vi "HFRR ADV v03 new software.vi"() -> ()   [LabVIEW 2025] (continued)
                      n2721 = Fract/Exp String To Number(string=w3763) -> (number=→"AVP 2":dbl)  [unwired: 3 in, 1 out]
                    }
                    frame 12 {
                      n2722 = Fract/Exp String To Number(string=w3765) -> (number=→"HCF 2":dbl)  [unwired: 3 in, 1 out]
                    }
                    frame 13 {
                      n2723 = Fract/Exp String To Number(string=w3767) -> (number=→"WS1.4 2":dbl)  [unwired: 3 in, 1 out]
                    }
                    frame 14, Default {
                    }
                  }
                }
              }
              frame #2 {
              }
            }
            n2724 = local write "OK Button 16"(FALSE ("OK Button 13")) -> ()
          }
        }
        n2725 = Index Array(array=w3411, index="Select Printer 3") -> (element=w3413:string)
        "Selected Printer" <- w3413
        n2726 = case shown="True" w3408 {
          frame False {
          }
          frame True {
            n2727 = flat-sequence {
              frame #0 {
              }
              frame #1 {
                n2728 = Wait (ms)(milliseconds to wait=u32 100) -> ()  [unwired: 1 out]
              }
              frame #2 {
                n2729 = local write "OK Button 16"(FALSE ("Print 3")) -> ()
              }
            }
          }
        }
        n2730 = case shown="True" "Print" {
          tunnel: w3413 -> [_ w3705]
          frame False {
          }
          frame True {
            (unwired) i16 6 ("width (-)")
            (unwired) "TESTED BY : "
            (unwired) "TESTED DATE :"
            (unwired) "SAMPLE ID : "
            (unwired) "SAMPLE DESIGN : "
            w3663 = "\r"
            w3680 = "\r"
            # "add image"
            n2731 = local read "Sample ID"() -> (w3653:string)
            n2732 = local read "Tested by"() -> (w3656:string)
            n2733 = local read "String 34"() -> (w3643:string)
            n2734 = local read "String 45"() -> (w3623:string)
            n2735 = local read "String 35"() -> (w3638:string)
            n2736 = local read "String 37"() -> (w3636:string)
            n2737 = local read "String 32"() -> (w3658:string)
            n2738 = local read "String 36"() -> (w3633:string)
            n2739 = local read "String 31"() -> (w3657:string)
            n2740 = local read "Test Date"() -> (w3654:string)
            n2741 = local read "String 33"() -> (w3659:string)
            n2742 = local read "String 38"() -> (w3629:string)
            n2743 = local read "String 39"() -> (w3626:string)
            n2744 = local write "Print"(FALSE ("Print FF")) -> ()
            n2745 = local read "S 39"() -> (w3641:string)
            n2746 = local read "S 38"() -> (w3648:string)
            n2747 = local read "Temperature before test 2"() -> (w3679:dbl)
            n2748 = local read "Temperature after test 2"() -> (w3669:dbl)
            n2749 = local read "Humidity before test 2"() -> (w3694:dbl)
            n2750 = local read "Humidity after test 2"() -> (w3678:dbl)
            n2751 = local read "MWSD 2"() -> (w3683:dbl)
            n2752 = local read "WS1.4 2"() -> (w3661:dbl)
            n2753 = Concatenate Strings("2)" ("string"), w3643) -> (w3644:string)
            n2754 = Concatenate Strings("3)" ("string"), w3641) -> (w3642:string)
            n2755 = Concatenate Strings("1)" ("string"), w3648) -> (w3647:string)
            n2756 = Concatenate Strings("4)" ("string"), w3638) -> (w3639:string)
            n2757 = Concatenate Strings("5)" ("string"), w3636) -> (w3635:string)
            n2758 = Concatenate Strings("6)" ("string"), w3633) -> (w3632:string)
            n2759 = Concatenate Strings("7)" ("string"), w3629) -> (w3630:string)
            n2760 = Concatenate Strings("8)" ("string"), w3626) -> (w3627:string)
            n2761 = local read "HCF 2"() -> (w3665:dbl)
            n2762 = local read "AVP 2"() -> (w3682:dbl)
            n2763 = local read "s.NO"() -> (w3624:string)
            n2764 = call <vilib>:"New Report.vi"("report type"=enum16{"Standard Report", "HTML"}."Standard Report") -> ("report out"=w3703:refnum<class "NI_report.lvclass">, "error out"=w3702:errorcluster)  [unwired: 13 in]
            n2765 = local read "TITTLE"() -> (w3655:string)
            n2766 = Concatenate Strings(w3680, w3623, w3624, w3680, w3658, w3653, w3680, w3657, w3654, w3680, w3659, w3656, w3680) -> (w3673:string)
            "test by" <- w3673
            n2767 = Number To Fractional String(number=w3679, width (-)=i16 6, precision (6)=i16 2) -> (F-format string=w3668:string)  [unwired: 1 in]
            n2768 = Number To Fractional String(number=w3678, width (-)=i16 6, precision (6)=i16 2) -> (F-format string=w3681:string)  [unwired: 1 in]
            n2769 = Number To Fractional String(number=w3694, width (-)=i16 6, precision (6)=i16 2) -> (F-format string=w3699:string)  [unwired: 1 in]
            n2770 = Number To Fractional String(number=w3683, width (-)=i16 6, precision (6)=i16 2) -> (F-format string=w3685:string)  [unwired: 1 in]
            n2771 = Number To Fractional String(number=w3669, width (-)=i16 6, precision (6)=i16 2) -> (F-format string=w3670:string)  [unwired: 1 in]
            n2772 = Number To Fractional String(number=w3682, width (-)=i16 6, precision (6)=i16 2) -> (F-format string=w3684:string)  [unwired: 1 in]
            n2773 = Number To Fractional String(number=w3665, width (-)=i16 6, precision (6)=i16 2) -> (F-format string=w3664:string)  [unwired: 1 in]
            n2774 = Number To Fractional String(number=w3661, precision (6)=i16 2) -> (F-format string=w3660:string)  [unwired: 2 in]
            n2775 = call-dynamic "Set Report Header Text.vi"("report in"=w3703, "center header text"=w3655, "error in (no error)"=w3702) -> ("report out"=w3674:refnum<class "NI_report.lvclass">, "error out"=w3675:errorcluster)  [unwired: 11 in]
            n2776 = Concatenate Strings(w3663, w3647, w3699, w3663, w3644, w3668, w3663, w3642, w3681, w3663, w3639, w3670, w3663, w3635, w3685, w3663, w3632, w3684, w3663, w3630, w3664, w3663, w3627, w3660) -> (w3651:string)
            "export 2" <- w3651
            n2777 = call-poly <vilib>:"Append Report Text.vi"("report in"=w3674, "text"=w3673, "error in (no error)"=w3675) -> ("report out"=w3677:refnum<class "NI_report.lvclass">, "error out"=w3676:errorcluster)  [unwired: 9 in, 2 out]
            n2778 = local read "test by"() -> (w3650:string)
            n2779 = local read "TITTLE"() -> (w3652:string)
            n2780 = call-poly <vilib>:"Append Report Text.vi"("report in"=w3677, "error in (no error)"=w3676) -> ("report out"=w3698:refnum<class "NI_report.lvclass">, "error out"=w3696:errorcluster)  [unwired: 10 in, 2 out]
            n2781 = Concatenate Strings(w3652, w3651, w3650) -> (→"output":string)
            n2782 = call-poly <vilib>:"Append Report Text.vi"("report in"=w3698, "text"=w3651, "error in (no error)"=w3696) -> ("report out"=w3697:refnum<class "NI_report.lvclass">, "error out"=w3695:errorcluster)  [unwired: 9 in, 2 out]
            n2783 = call-dynamic "Print Report.vi"("report in"=w3697, "printer name (default)"=w3705, "error in (no error)"=w3695) -> ("report out"=w3707:refnum<class "NI_report.lvclass">, "error out"=w3708:errorcluster)  [unwired: 11 in]
            n2784 = call-dynamic "Dispose Report.vi"("report in"=w3707, "error in (no error)"=w3708) -> ()  [unwired: 13 in, 1 out]
          }
        }
        n2785 = case shown="True" "Print 2" {
          frame False {
          }
          frame True {
            n2786 = flat-sequence {
              frame #0 {
                n2787 = local read "s.NO"() -> (→"s.NO 2":string)
                n2788 = Wait (ms)(milliseconds to wait=u32 20) -> ()  [unwired: 1 out]
                n2789 = local read "Sample ID  3"() -> (→"Sample ID  6":string)
                n2790 = local read "Sample ID  4"() -> (→"Sample ID  7":string)
                n2791 = local read "Sample ID"() -> (→"Sample ID  2":string)
                n2792 = local read "Tested by"() -> (→"Tested by 2":string)
                n2793 = local read "Test Date"() -> (→"Test Date 2":string)
                n2794 = local read "Humidity after test 3"() -> (→"Humidity after test 4":dbl)
                n2795 = local read "Ref A Test Date :"() -> (→"TITTLE 4":string)
                n2796 = local read "Temperature before test 3"() -> (w3530:dbl)
                n2797 = local read "Temperature before test 3"() -> (→"Temperature after test 5":dbl)
                n2798 = local read "Temperature after test 3"() -> (→"Temperature after test 4":dbl)
                n2799 = local read "Humidity before test 3"() -> (→"Humidity before test 4":dbl)
                n2800 = local write "Temperature before test 3"(w3530) -> ()
                n2801 = local read "image data"() -> (w3521:T11)
                n2802 = String To Path(string="C:\\LAB-IQ\\im\\Temp_resized.jpg") -> (path=w3522:path)
                "path 2" <- w3522
                n2803 = call <vilib>:"Write JPEG File.vi"("image data"=w3521, "path to JPEG file"=w3522) -> ()  [unwired: 8 in, 2 out]
                "Ref A Test Date :" <- "Ref A Test Date :"
                "Ref B Test Date :" <- "Ref B Test Date :"
                "Ref B Scar Value :" <- "Ref B Scar Value :"
                "Ref A Scar Value :" <- "Ref A Scar Value :"
              }
              frame #1 {
                (unwired) HTML_Report_Image_Alignment."MIDDLE" ("alignment (default)")
                w3558 = u16 0 items=["portrait", "landscape"] ("orientation (portrait)")
                (unwired) HTML_Report_Image_Alignment."ABSMIDDLE" ("alignment (default)")
                (unwired) "TESTED BY : "
                (unwired) "TESTED DATE :"
                (unwired) "SAMPLE ID : "
                (unwired) "SAMPLE DESIGN : "
                w3591 = "\r"
                # "add image"
                n2804 = Wait (ms)(milliseconds to wait=u32 20) -> ()  [unwired: 1 out]
                n2805 = local read "Sample ID  2"() -> (w3584:string)
                n2806 = local read "Wear Scar X"() -> (w3556:dbl)
                "Length ( microns ) 2" <- w3556
                n2807 = local read "Wear Scar Y"() -> (w3555:dbl)
                "Wear Scar Y ( microns ) :" <- w3555
                n2808 = local read "Test Date 2"() -> (w3585:string)
                n2809 = local read "Tested by 2"() -> (w3586:string)
                n2810 = local read "String 46"() -> (w3582:string)
                n2811 = local read "String 48"() -> (w3588:string)
                n2812 = local read "String 47"() -> (w3587:string)
                n2813 = local read "String 49"() -> (w3589:string)
                n2814 = local read "String 10"() -> (w3542:string)
                n2815 = local read "s.NO 2"() -> (w3583:string)
                n2816 = Add(x=w3556, y=w3555) -> (x+y=w3554:dbl)
                n2817 = call <vilib>:"New Report.vi"("report type"=enum16{"Standard Report", "HTML"}."HTML") -> ("report out"=w3562:refnum<class "NI_report.lvclass">, "error out"=w3560:errorcluster)  [unwired: 13 in]
                n2818 = Concatenate Strings(w3591, w3582, w3583, w3591, w3588, w3584, w3591, w3587, w3585, w3591, w3589, w3586, w3591) -> (→"test by 2":string)
                n2819 = Concatenate Strings("C:\\LAB-IQ\\Data\\" ("string"), w3542, ".jpg" ("string")) -> ()  [unwired: 1 out]
                n2820 = Divide(x=w3554, y=2.0) -> (x/y=→"Mean Wear ( microns) :":dbl)
                n2821 = call-dynamic "Set Report Orientation.vi"("report in"=w3562, "orientation (portrait)"=w3558, "error in (no error)"=w3560) -> ("report out"=w3561:refnum<class "NI_report.lvclass">, "error out"=w3559:errorcluster)  [unwired: 11 in]
                n2822 = for {
                  N: 5 -> [_]
                  tunnel: w3561 -> [w3612]
                  tunnel: [w3611] -> w3540
                  tunnel: w3559 -> [w3610]
                  tunnel: [w3609] -> w3539
                  n2823 = call-dynamic "Set Report Tab Width.vi"("report in"=w3612, "error in (no error)"=w3610) -> ("report out"=w3611:refnum<class "NI_report.lvclass">, "error out"=w3609:errorcluster)  [unwired: 12 in]
                }
                n2824 = local read "TITTLE"() -> (w3557:string)
                n2825 = call-dynamic "Set Report Header Text.vi"("report in"=w3540, "center header text"=w3557, "error in (no error)"=w3539) -> ("report out"=w3578:refnum<class "NI_report.lvclass">, "error out"=w3577:errorcluster)  [unwired: 11 in]
                n2826 = for {
                  N: 1 -> [_]
                  tunnel: [w3616] -> w3564
                  tunnel: [w3615] -> w3563
                  tunnel: w3578 -> [w3614]
                  tunnel: w3577 -> [w3613]
                  n2827 = call-dynamic "New Report Line.vi"("report in"=w3614, "error in (no error)"=w3613) -> ("report out"=w3616:refnum<class "NI_report.lvclass">, "error out"=w3615:errorcluster)  [unwired: 12 in]
                }
                n2828 = for {
                  N: 2 -> [_]
                  tunnel: [w3608] -> w3570
                  tunnel: [w3607] -> w3569
                  tunnel: w3564 -> [w3606]
                  tunnel: w3563 -> [w3605]
                  n2829 = call-dynamic "New Report Line.vi"("report in"=w3606, "error in (no error)"=w3605) -> ("report out"=w3608:refnum<class "NI_report.lvclass">, "error out"=w3607:errorcluster)  [unwired: 12 in]
                }
                n2830 = for {
                  N: 25 -> [_]
                  tunnel: w3570 -> [w3604]
                  tunnel: w3569 -> [w3602]
                  tunnel: [w3603] -> w3573
                  tunnel: [w3601] -> w3572
                  n2831 = call-dynamic "Set Report Tab Width.vi"("report in"=w3604, "error in (no error)"=w3602) -> ("report out"=w3603:refnum<class "NI_report.lvclass">, "error out"=w3601:errorcluster)  [unwired: 12 in]
                }
                n2832 = control-ref of="Tab Control 9"() -> (w3568:refnum<vi>)
                n2833 = call-dynamic "Append Control Image to Report.vi"("report in"=w3573, "alignment (default)"=HTML_Report_Image_Alignment."ABSMIDDLE", "ctrl reference"=w3568, "error in (no error)"=w3572) -> ("report out"=w3567:refnum<class "NI_report.lvclass">, "error out"=w3566:errorcluster)  [unwired: 8 in, 2 out]
                n2834 = for {
                  N: 3 -> [_]
                  tunnel: [w3600] -> w3551
                  tunnel: [w3599] -> w3550
                  tunnel: w3567 -> [w3598]
                  tunnel: w3566 -> [w3597]
                  n2835 = call-dynamic "New Report Line.vi"("report in"=w3598, "error in (no error)"=w3597) -> ("report out"=w3600:refnum<class "NI_report.lvclass">, "error out"=w3599:errorcluster)  [unwired: 12 in]
                }
                n2836 = for {
                  N: 100 -> [_]
                  tunnel: w3551 -> [w3596]
                  tunnel: w3550 -> [w3594]
                  tunnel: [w3595] -> w3547
                  tunnel: [w3593] -> w3545
                  n2837 = call-dynamic "Set Report Tab Width.vi"("report in"=w3596, "error in (no error)"=w3594) -> ("report out"=w3595:refnum<class "NI_report.lvclass">, "error out"=w3593:errorcluster)  [unwired: 12 in]
                }
                n2838 = String To Path(string="C:\\LAB-IQ\\im\\Temp_resized.jpg") -> (path=w3537:path)
                n2839 = call-poly <vilib>:"Append Image to Report.vi"("report in"=w3547, "path or URL of image"=w3537, "error in (no error)"=w3545) -> ("report out"=w3546:refnum<class "NI_report.lvclass">, "error out"=w3544:errorcluster)  [unwired: 9 in, 2 out]
                n2840 = call-poly <vilib>:"Open HTML Report in Browser.vi"("report in"=w3546, "error in (no error)"=w3544) -> ("report out"=w3581:refnum<class "NI_report.lvclass">, "error out"=w3580:errorcluster)  [unwired: 11 in, 1 out]
                n2841 = call-dynamic "Dispose Report.vi"("report in"=w3581, "error in (no error)"=w3580) -> ()  [unwired: 13 in, 1 out]
              }
              frame #2 {
              }
              frame #3 {
                n2842 = disable-structure shown="Disabled" {
                  frame Disabled {
                    n2843 = local read "String 10"() -> (w3621:string)
                    n2844 = Concatenate Strings("C:\\LAB-IQ-NXT\\Data\\" ("string"), w3621, ".jpg" ("string")) -> (w3619:string)
                    n2845 = String To Path(string=w3619) -> (path=w3618:path)
                    n2846 = Delete(path (use dialog)=w3618) -> ()  [unwired: 4 in, 3 out]
                  }
                  frame Enabled {
                  }
                }
                n2847 = local write "Print 2"(FALSE ("Print")) -> ()
              }
            }
          }
        }
      }
    }
    n2848 = property on="SetTemp" class="DigNum (strict)"("Disabled"=w1582) -> ()  [unwired: 2 in, 2 out]
    n2849 = Multiply(x=w1572, y=w1574) -> (x*y=w1573:dbl)
    n2850 = local read "MWSD"() -> (w1571:dbl)
    n2851 = Add(x=w1573, y=w1571) -> (x+y=→"WS1.4":dbl)
    n2852 = Wait (ms)(milliseconds to wait=u32 50) -> ()  [unwired: 1 out]
    n2853 = Wait (ms)(milliseconds to wait=u32 50) -> ()  [unwired: 1 out]
    n2854 = local read "Quit"() -> (w1570:bool)
  }
  n2855 = VISA Close(VISA resource name=w52, error in (no error)=w51) -> (error out=w49:errorcluster)
  n2856 = call <vilib>:"Clear Errors.vi"("error in (no error)"=w49) -> ()  [unwired: 5 in, 2 out]
  n2857 = VISA Close(VISA resource name=w37, error in (no error)=w36) -> ()  [unwired: 1 out]
  n2858 = while {
    tunnel: [w3780] -> w46
    shift-right: [w3773] -> _
    shift-left: 0.0 -> [w3776]
    shift-right: [w3772] -> _
    shift-left: 0.0 -> [w3775]
    shift-right: [w3771] -> _
    shift-left: 400.0 ("vc_cmd") -> [w3774]
    stop <- w3780 stop-if-true
    # "PID LOGIC"
    n2859 = local read "RUN"() -> (w3778:bool)
    n2860 = local read "Auto Start Test"() -> (w3777:bool)
    n2861 = local read "START TEMP"() -> (w3769:bool)
    n2862 = Or(x=w3778, y=w3777) -> (x .or. y?=w3779:bool)
    n2863 = And(x=w3779, y=w3769) -> (x .and. y?=w3770:bool)
    n2864 = Wait (ms)(milliseconds to wait=u32 20) -> ()  [unwired: 1 out]
    n2865 = case shown="True" w3770 {
      tunnel: [400.0 ("out_vc_cmd") w3798] -> w3771
      tunnel: [w3783 w3800] -> w3772
      tunnel: [w3783 w3799] -> w3773
      tunnel: w3776 -> [_ w3787]
      tunnel: w3775 -> [_ w3786]
      tunnel: w3774 -> [_ w3785]
      frame False {
        w3783 = 0.0 ("error_out")
      }
      frame True {
        n2866 = local read "measured_stroke"() -> (w3788:dbl)
        n2867 = local read "Set Strk"() -> (w3797:dbl)
        n2868 = formula code="// Zero-Hardcode Explicit Positional-Form PID Engine\n// Inputs: target_stroke, measured_stroke, dt, prev_error, integral_accumulator_in, prev_vc_cmd\n//         kp, ki, kd, max_step_change, max_amplitude, min_amplitude, startup_cmd\n// Outputs: vc_cmd, error_out, out_error, integral_accumulator_out, out_vc_cmd\n\n// 1. Calculate Tracking Error\nfloat current_error = target_stroke - measured_stroke;\nerror_out = current_error;\n\n// 2. Compute Proportional Term\nfloat p_term = kp * current_error;\n\n// 3. Compute Derivative Term\nfloat d_term = 0.0;\nif (dt > 0.0) {\n    d_term = kd * ((current_error - prev_error) / dt);\n}\n\n// 4. Update and Accumulate Integral Term\nfloat current_integral = integral_accumulator_in + (current_error * dt);\nfloat i_term = ki * current_integral;\n\n// 5. Calculate Ideal Target Command\nfloat ideal_command = startup_cmd + p_term + i_term + d_term;\n\n// 6. Anti-Windup Protection (Back-calculation method)\nif (ideal_command > max_amplitude) {\n    float excess = ideal_command - max_amplitude;\n    if (ki > 0.0) {\n        current_integral -= excess / ki;\n    }\n    ideal_command = max_amplitude;\n} else if (ideal_command < min_amplitude) {\n    float excess = ideal_command - min_amplitude;\n    if (ki > 0.0) {\n        current_integral -= excess / ki;\n    }\n    ideal_command = min_amplitude;\n}\n\n// 7. Apply Loop Rate Limiting (Protects voice coil from large voltage steps)\nfloat raw_adjustment = ideal_command - prev_vc_cmd;\n\nif (raw_adjustment > max_step_change) {\n    raw_adjustment = max_step_change;\n} else if (raw_adjustment < -max_step_change) {\n    raw_adjustment = -max_step_change;\n}\n\nfloat next_vc_cmd = prev_vc_cmd + raw_adjustment;\n\n// Final Output Safety Safeguard Clamping\nif (next_vc_cmd > max_amplitude) {\n    next_vc_cmd = max_amplitude;\n} else if (next_vc_cmd < min_amplitude) {\n    next_vc_cmd = min_amplitude;\n}\n\n// 8. Map to Shift Registers for memory persistence\nvc_cmd = next_vc_cmd;\nout_error = current_error;                     \nintegral_accumulator_out = current_integral;  \nout_vc_cmd = next_vc_cmd;"("target_stroke"=w3797, "measured_stroke"=w3788, "dt"="dt", "integral_accumulator_in"=w3786, "prev_error"=w3787, "prev_vc_cmd"=w3785, "kp"="kp", "ki"="ki", "kd"="kd", "max_step_change"="max_step_change", "max_amplitude"="max_amplitude", "min_amplitude"="min_amplitude", "startup_cmd"="startup_cmd") -> ("vc_cmd"=w3804:dbl, "out_error"=w3799:dbl, "integral_accumulator_out"=w3800:dbl, "out_vc_cmd"=w3798:dbl)  [unwired: 1 out]
        "output Vpp" <- w3804
        n2869 = Number To Fractional String(number=w3804, precision (6)=i16 1) -> (F-format string=w3802:string)  [unwired: 2 in]
        n2870 = Concatenate Strings("V" ("string"), w3802) -> (w3784:string)
        n2871 = local write "Command"(w3784) -> ()
        "prev_error" <- w3787
        "integral_accumulator_in" <- w3786
        "prev_vc_cmd" <- w3785
      }
    }
    n2872 = local read "Quit"() -> (w3780:bool)
  }
  n2873 = Or(x=w42, y=w41) -> (x .or. y?=w43:bool)
  n2874 = Or(x=w39, y=w43) -> (x .or. y?=w48:bool)
  n2875 = control-ref of="new picture"() -> ()  [unwired: 1 out]
  n2876 = Or(x=w54, y=w48) -> (x .or. y?=w45:bool)
  n2877 = Or(x=w45, y=w46) -> (x .or. y?=w40:bool)
  n2878 = while {
    tunnel: [w3805] -> w53
    i -> [w3812]
    stop <- w3805 stop-if-true
    n2879 = local read "Quit"() -> (w3805:bool)
    n2880 = Equal To 0?(x=w3812) -> (x = 0?=w3810:bool)
    n2881 = call "Elapsed Time3"("Time Target (s)"=45.0, "Auto Reset"=TRUE) -> ("Time has Elapsed"=w3809:bool)  [unwired: 10 in, 7 out]
    n2882 = Wait (ms)(milliseconds to wait=u32 50) -> ()  [unwired: 1 out]
    n2883 = Or(x=w3809, y=w3810) -> (x .or. y?=w3811:bool)
    n2884 = case shown="True" w3811 {
      frame False {
      }
      frame True {
        n2885 = call <vilib>:"System Exec.vi"("run minimized? (F)"=TRUE, "error in (no error)"="error in (no error)", "command line"="powercfg.exe -change -monitor-timeout-ac 0") -> ("error out"=w3823:errorcluster)  [unwired: 5 in, 3 out]
        n2886 = call <vilib>:"System Exec.vi"("run minimized? (F)"=TRUE, "error in (no error)"=w3823, "command line"="powercfg.exe -change -disk-timeout-ac 0") -> ("error out"=w3822:errorcluster)  [unwired: 5 in, 3 out]
        n2887 = call <vilib>:"System Exec.vi"("run minimized? (F)"=TRUE, "error in (no error)"=w3822, "command line"="powercfg.exe -change -standby-timeout-ac 0") -> ("error out"=w3821:errorcluster)  [unwired: 5 in, 3 out]
        n2888 = call <vilib>:"System Exec.vi"("run minimized? (F)"=TRUE, "error in (no error)"=w3821, "command line"="powercfg.exe -change -hibernate-timeout-ac 0") -> ("error out"=w3820:errorcluster)  [unwired: 5 in, 3 out]
        n2889 = call <vilib>:"Simple Error Handler.vi"("error in (no error)"=w3820) -> ("error out"=w3826:errorcluster)  [unwired: 4 in, 4 out]
        n2890 = call <vilib>:"Clear Errors.vi"("error in (no error)"=w3826) -> ("error out"=→"error out":errorcluster)  [unwired: 5 in, 1 out]
      }
    }
  }
  n2891 = Compound Arithmetic op=OR(w56, w40, w53) -> (w55:bool)
  n2892 = flat-sequence {
    tunnel: w55 -> [_]
    tunnel: [w3828] -> w17
    tunnel: w17 -> [_]
    frame #0 {
      n2893 = call "CLOSE CONNECTION.vi"() -> ("error out"=w3828:errorcluster)  [unwired: 11 in]
    }
    frame #1 {
      n2894 = Quit LabVIEW(quit? (T)=TRUE) -> ()
      n2895 = local write "Quit"(FALSE ("EXIT")) -> ()
    }
  }
  n2896 = property on="Heater Button" class="Bool (strict)"("Visible"=TRUE) -> ()  [unwired: 2 in, 2 out]
  n2897 = disable-structure shown="Disabled" {
    disable-tunnel: _ -> [w3834 _]
    disable-tunnel: _ -> [w3831 _]
    disable-tunnel: _ -> [w3832 _]
    frame Disabled {
      n2898 = disable-structure shown="Disabled" {
        disable-tunnel: [w3841 _] -> w3833
        frame Disabled {
          n2899 = while {
            shift-right: [w3883] -> w3839
            shift-left: errorcluster {"status"=TRUE, "code"=0, "source"="Init"} ("error out") -> [w3848]
            shift-right: [w3882] -> w3838
            shift-left: _ -> [w3849]
            shift-right: [w3881] -> _
            shift-left: "" -> [w3880]
            tunnel: [w3842] -> w3841
            shift-right: ["Set Rh"] -> _
            shift-left: 0.0 ("Set Rh") -> [w3874]
            tunnel: [w3851] -> _
            i -> [w3851]
            stop <- w3842 stop-if-true
            n2900 = flat-sequence {
              tunnel: w3848 -> [w3886]
              tunnel: [w3886] -> w3847
              frame #0 {
                n2901 = Wait (ms)(milliseconds to wait=u32 200) -> ()  [unwired: 1 out]
              }
            }
            n2902 = local read "Com Port 3"() -> (w3850:refnum<visa-resource-name>)
            n2903 = local read "Humidity Str Rec"() -> (w3852:string)
            n2904 = Not Equal?(x="Set Rh", y=w3874) -> (x != y?=w3879:bool)
            n2905 = Number To Decimal String(number="Set Rh") -> (decimal integer string=w3877:string)  [unwired: 1 in]
            n2906 = Not Equal?(x=w3850, y=w3849) -> (x != y?=w3845:bool)
            n2907 = Concatenate Strings("#setPoint00" ("string"), w3877) -> (w3878:string)
            n2908 = case shown="False" w3879 {
              tunnel: w3878 -> [_ w3898]
              frame False {
                n2909 = local read "Humidity"() -> (w3895:bool)
                n2910 = case shown="True" w3895 {
                  frame False {
                    n2911 = local write "Humidity Str Send"("stop" ("Humidity Str Send")) -> ()
                  }
                  frame True {
                    n2912 = local write "Humidity Str Send"("start" ("Humidity Str Send")) -> ()
                  }
                }
              }
              frame True {
                n2913 = local write "Humidity Str Send"(w3898) -> ()
              }
            }
            n2914 = Or(x=w3845) -> (y=w3843:bool, x .or. y?=w3844:bool)
            n2915 = String Subset(string=w3852, offset (0)=7) -> (substring=w3867:string)  [unwired: 1 in]
            n2916 = Match Pattern(string=w3852, regular expression="?") -> (offset past match=w3870:i32)  [unwired: 1 in, 3 out]
            n2917 = Match Pattern(string=w3852, regular expression="v") -> (offset past match=w3873:i32)  [unwired: 1 in, 3 out]
            n2918 = case shown="True" w3844 {
              tunnel: w3847 -> [w3884 _]
              tunnel: [w3884 errorcluster {"status"=TRUE, "code"=0, "source"="Init"} ("error out")] -> w3846
              frame False {
              }
              frame True {
              }
            }
            n2919 = Equal?(x=w3870, y=-1) -> (x = y?=w3854:bool)
            n2920 = Match Pattern(string=w3867, regular expression="g") -> (after substring=w3868:string, offset past match=w3859:i32)  [unwired: 1 in, 2 out]
            n2921 = Match Pattern(string=w3867, regular expression="y") -> (after substring=w3866:string, offset past match=w3860:i32)  [unwired: 1 in, 2 out]
            n2922 = Greater?(x=w3860, y=w3859) -> (0:w3865:bool)
            n2923 = Greater Or Equal To 0?(x=w3860) -> (x >= 0?=w3857:bool)
            n2924 = Greater Or Equal To 0?(x=w3859) -> (x >= 0?=w3858:bool)
            n2925 = Or(x=w3857, y=w3858) -> (x .or. y?=w3856:bool)
            n2926 = Greater Or Equal To 0?(x=w3873) -> (x >= 0?=w3855:bool)
            n2927 = Select(t=w3866, s=w3865, f=w3868) -> (s? t:f=w3861:string)
            n2928 = case shown="Error" w3846 {
              selector: w3846 -> [w3911 w3957]
              tunnel: [w3909 w3950] -> w3883
              tunnel: w3849 -> [w3912 w3956]
              tunnel: [w3910 w3959] -> w3882
              tunnel: w3880 -> [w3899 w3958]
              tunnel: [w3906 w3958] -> w3881
              frame No Error {
                n2929 = call "Elapsed Time7"() -> ("Time has Elapsed"=w3905:bool)  [unwired: 12 in, 7 out]
                n2930 = Not Equal?(x="Humidity Str Send", y=w3899) -> (x != y?=w3901:bool)
                n2931 = Or(x=w3901, y=w3905) -> (x .or. y?=w3904:bool)
                n2932 = Select(t="Humidity Str Send", s=w3901, f="vals" ("regular expression")) -> (s? t:f=w3900:string)
                n2933 = Or(x=w3904, y="Send") -> (x .or. y?=w3908:bool)
                n2934 = case shown="True" w3908 {
                  tunnel: [w3915 w3920] -> w3909
                  tunnel: w3912 -> [w3914 w3928]
                  tunnel: w3911 -> [w3915 w3927]
                  tunnel: [w3914 w3921] -> w3910
                  tunnel: w3900 -> [_ w3926]
                  tunnel: [w3913 w3917] -> w3906
                  tunnel: "Humidity Str Send" -> [_ w3918]
                  tunnel: w3901 -> [_ w3919]
                  tunnel: w3899 -> [w3913 w3916]
                  frame False {
                  }
                  frame True {
                    n2935 = flat-sequence {
                      tunnel: w3928 -> [w3936]
                      tunnel: w3927 -> [w3935]
                      tunnel: w3926 -> [w3932]
                      tunnel: [w3934] -> w3925
                      tunnel: [w3933] -> w3924
                      tunnel: w3925 -> [w3939]
                      tunnel: w3924 -> [w3938]
                      tunnel: [w3939] -> w3923
                      tunnel: [w3938] -> w3922
                      tunnel: w3923 -> [w3946]
                      tunnel: w3922 -> [w3945]
                      tunnel: [w3944] -> w3921
                      tunnel: [w3943] -> w3920
                      frame #0 {
                        n2936 = local write "Ser Led"(TRUE ("Boolean 4")) -> ()
                        n2937 = Concatenate Strings(w3932, "\r") -> (w3931:string)
                        n2938 = VISA Write(VISA resource name=w3936, write buffer=w3931, error in (no error)=w3935) -> (VISA resource name out=w3934:refnum<visa-resource-name>, error out=w3933:errorcluster)  [unwired: 1 out]
                      }
                      frame #1 {
                        n2939 = Wait (ms)(milliseconds to wait="wait") -> ()  [unwired: 1 out]
                      }
                      frame #2 {
                        w3941 = FALSE ("Send")
                        n2940 = property class="Instr"(reference=w3946, error in=w3945) -> (reference out=w3947:refnum<visa-resource-name>, error out=w3948:errorcluster, "Serial Settings:Number of Bytes at Serial Port"=w3940:u32)
                        n2941 = local write "Send"(w3941) -> ()
                        n2942 = local write "Ser Led"(w3941) -> ()
                        n2943 = VISA Read(VISA resource name=w3947, byte count=w3940, error in (no error)=w3948) -> (VISA resource name out=w3944:refnum<visa-resource-name>, read buffer=→"Humidity Str Rec":string, error out=w3943:errorcluster)  [unwired: 1 out]
                      }
                    }
                    n2944 = Select(t=w3918, s=w3919, f=w3916) -> (s? t:f=w3917:string)
                  }
                }
              }
              frame Error {
                w3964 = u16 0 items=["None"=0, "XON/XOFF"=1, "RTS/CTS"=2, "DTR/DSR"=4] ("flow control")
                w3960 = u16 0 items=["None", "Odd", "Even", "Mark", "Space"] ("parity")
                w3963 = u16 10 items=["1.0"=10, "1.5"=15, "2.0"=20] ("stop bits")
                n2945 = VISA Close(VISA resource name=w3956, error in (no error)=w3957) -> (error out=w3955:errorcluster)
                n2946 = local write "humid"("" ("humid")) -> ()
                n2947 = local write "Humidity Str Rec"("" ("Humidity Str Rec")) -> ()
                n2948 = call <vilib>:"Clear Errors.vi"("error in (no error)"=w3955) -> ("error out"=w3954:errorcluster)  [unwired: 5 in, 1 out]
                n2949 = local read "Com Port 3"() -> (w3953:refnum<visa-resource-name>)
                n2950 = call-poly "VISA Configure Serial Port"("VISA resource name"=w3953, "timeout (10sec)"=u32 1000, "termination char\n(0xA = '\\n' = LF)"=u8 10 ("termination char\n(0xA = '\\n' = LF)"), "Enable Termination\nChar (T)"=FALSE ("Enable Termination Char (T)"), "data bits (8)"=u16 8 ("data bits"), "parity (0:none)"=w3960, "error in (no error)"=w3954, "stop bits (10: 1 bit)"=w3963, "flow control (0:none)"=w3964) -> ("VISA resource name out"=w3959:refnum<visa-resource-name>, "baud rate (9600)"=w3951:u32, "error out"=w3950:errorcluster)  [unwired: 4 in]
              }
            }
            n2951 = Compound Arithmetic op=AND(w3855, w3854, w3856) -> (w3853:bool)
            n2952 = case shown="True" w3853 {
              tunnel: w3852 -> [_ _]
              tunnel: w3861 -> [_ w3891]
              frame False {
              }
              frame True {
                w3889 = " " ("regular expression")
                n2953 = Match Pattern(string=w3891, regular expression=" ") -> (after substring=w3893:string)  [unwired: 1 in, 3 out]
                n2954 = Match Pattern(string=w3893, regular expression=w3889) -> (before substring=→"humid":string, after substring=w3890:string)  [unwired: 1 in, 2 out]
                n2955 = Match Pattern(string=w3890, regular expression=w3889) -> (before substring=→"temp_@Rh sensor":string)  [unwired: 1 in, 3 out]
              }
            }
            n2956 = local read "Quit"() -> (w3842:bool)
          }
          n2957 = VISA Close(VISA resource name=w3838, error in (no error)=w3839) -> (error out=w3835:errorcluster)
          n2958 = call <vilib>:"Clear Errors.vi"("error in (no error)"=w3835) -> ()  [unwired: 5 in, 2 out]
        }
        frame Enabled {
        }
      }
    }
    frame Enabled {
    }
  }
  n2959 = while {
    tunnel: [w3971] -> _
    i -> [w3971]
    stop <- w3967 stop-if-true
    # "Langauage selection"
    n2960 = Equal?(x="Lan flag", y=22.0) -> ()  [unwired: 1 out]
    n2961 = disable-structure shown="Disabled" {
      frame Disabled {
        n2962 = stacked-sequence {
          frame #0 {
            n2963 = case shown="\"Russian\"" "Language Selection" {
              tunnel: [0 1] -> w3973
              frame "English", Default {
              }
              frame "Russian" {
              }
            }
            n2964 = for {
              N: 130 -> [_]
              tunnel: "Table" -> [w3982]
              tunnel: w3973 -> [w3981]
              i -> [w3980]
              n2965 = Index Array(array=w3982, index (row)=w3980, index (col)=w3981) -> (element=w3979:string)
              n2966 = case shown="123" w3980 {
                tunnel: w3979 -> [w3983 w3984 _ w3985 w3986 w3987 w3988 w3989 w3990 w3991 w3992 w3993 w3994 w3995 w3996 w3997 w3998 w3999 w4000 w4001 w4002 w4003 w4004 w4005 w4006 w4007 w4008 w4009 w4010 _ _ w4011 w4012 w4013 w4014 w4015 w4016 w4025 w4032 w4039 w4046 w4050 w4053 w4056 w4058 w4060 w4061 w4062 w4063 w4064 w4065 w4066 w4067 w4068 w4069 w4070 w4071 w4072 w4073 w4074 w4075 w4076 w4077 w4078 w4079 w4080 w4081 w4082 w4083 w4084 w4085 w4086 w4087 w4088 w4089 w4090 w4091 w4092 w4093 w4094 w4095 w4096 w4097 w4098 w4099 w4100 w4101 w4102 w4103 w4104 w4105 w4106 w4107 w4108 w4109 w4110 w4111 w4112 w4113 w4114 w4115 w4116 w4117 w4118 w4119 _ w4120 w4121 w4122 w4123 w4124 w4125 w4126 w4127 w4128 w4129 w4130 w4131 w4132 _ w4133 w4134 w4135 w4136 w4137 w4138 _]
                frame 0 {
                  n2967 = local write "S"(w3983) -> ()
                }
                frame 1 {
                  n2968 = local write "S 2"(w3984) -> ()
                }
                frame 2 {
                }
                frame 3 {
                  n2969 = local write "S 4"(w3985) -> ()
                }
                frame 4 {
                  n2970 = property on="FILE" class="Str"("Caption.Text"=w3986) -> ()  [unwired: 2 in, 2 out]
                }
                frame 5 {
                  n2971 = property on="Fuel Discription :" class="Str"("Caption.Text"=w3987) -> ()  [unwired: 2 in, 2 out]
                }
                frame 6 {
                  n2972 = property on="Remarks :" class="Str"("Caption.Text"=w3988) -> ()  [unwired: 2 in, 2 out]
                }
                frame 7 {
                  n2973 = property on="Save & Continue" class="Bool (strict)"("Boolean Text.Text"=w3989) -> ()  [unwired: 2 in, 2 out]
                }
                frame 8 {
                }
                frame 9 {
                  n2974 = property on="Set Hz" class="DigNum (strict)"("Caption.Text"=w3991) -> ()  [unwired: 2 in, 2 out]
                }
                frame 10 {
                  "String 3" <- w3992
                }
                frame 11 {
                  n2975 = property on="NORMAL LOAD" class="DigNum (strict)"("Caption.Text"=w3993) -> ()  [unwired: 2 in, 2 out]
                }
                frame 12 {
                  "String 5" <- w3994
                }
                frame 13 {
                  n2976 = property on="Set Temp" class="DigNum (strict)"("Caption.Text"=w3995) -> ()  [unwired: 2 in, 2 out]
                }
                frame 14 {
                  n2977 = local write "S 15"(w3996) -> ()
                }
                frame 15 {
                  n2978 = property on="Set Rh" class="DigNum (strict)"("Caption.Text"=w3997) -> ()  [unwired: 2 in, 2 out]
                }
                frame 16 {
                  "String 13" <- w3998
                  "String 26" <- w3998
                }
                frame 17 {
                  n2979 = local write "S 18"(w3999) -> ()
                }
                frame 18 {
                  "String 17" <- w4000
                }
                frame 19 {
                  n2980 = property on="test time" class="DigNum (strict)"("Caption.Text"=w4001) -> ()  [unwired: 2 in, 2 out]
                }
                frame 20 {
                  "String 18" <- w4002
                  "String 22" <- w4002
                }
                frame 21 {
                  n2981 = property on="Elapsed time" class="DigNum (strict)"("Caption.Text"=w4003) -> ()  [unwired: 2 in, 2 out]
                }
                frame 22 {
                  n2982 = property on="Samplingtime 2" class="DigNum (strict)"("Caption.Text"=w4004) -> ()  [unwired: 2 in, 2 out]
                }
                frame 23 {
                  "String 21" <- w4005
                }
                frame 24 {
                  n2983 = property on="Countdown" class="DigNum (strict)"("Caption.Text"=w4006) -> ()  [unwired: 2 in, 2 out]
                }
                frame 25 {
                  n2984 = property on="Countdown 2" class="DigNum (strict)"("Caption.Text"=w4007) -> ()  [unwired: 2 in, 2 out]
                }
                frame 26 {
                  n2985 = property on="Engage" class="Bool (strict)"("Boolean Text.Text"=w4008) -> ()  [unwired: 2 in, 2 out]
                }
                frame 27 {
                  n2986 = property on="Boolean  4" class="Bool (strict)"("Boolean Text.Text"=w4009) -> ()  [unwired: 2 in, 2 out]
                }
                frame 28 {
                  n2987 = property on="Test \nStatus" class="Bool (strict)"("Boolean Text.Text"=w4010) -> ()  [unwired: 2 in, 2 out]
                }
                frame 29 {
                }
                frame 30 {
                }
                frame 31 {
                }
                frame 32 {
                  n2988 = property on="RSTCOF" class="Bool"("Boolean Text.Text"=w4012) -> ()  [unwired: 2 in, 2 out]
                  n2989 = property on="RST FF" class="Bool"("Boolean Text.Text"=w4012) -> ()  [unwired: 2 in, 2 out]
                  n2990 = property on="RST TEMP" class="Bool"("Boolean Text.Text"=w4012) -> ()  [unwired: 2 in, 2 out]
                  n2991 = property on="RSTV1 3" class="Bool"("Boolean Text.Text"=w4012) -> ()  [unwired: 2 in, 2 out]
                  n2992 = property on="rstv2" class="Bool"("Boolean Text.Text"=w4012) -> ()  [unwired: 2 in, 2 out]
                  n2993 = property on="RSTV1 2" class="Bool"("Boolean Text.Text"=w4012) -> ()  [unwired: 2 in, 2 out]
                  n2994 = property on="RST CP" class="Bool"("Boolean Text.Text"=w4012) -> ()  [unwired: 2 in, 2 out]
                }
                frame 33 {
                  "S 61" <- w4013
                }
                frame 34 {
                  "String 23" <- w4014
                }
                frame 35 {
                  n2995 = property on="Rh Before" class="DigNum (strict)"("Caption.Text"=w4015) -> ()  [unwired: 2 in, 2 out]
                }
                frame 36 {
                  n2996 = Match Pattern(string=w4016, regular expression=",") -> (before substring=→"bs":string, after substring=→"as":string)  [unwired: 1 in, 2 out]
                  n2997 = property on="Rh After" class="DigNum (strict)"("Caption.Text"=w4016) -> ()  [unwired: 2 in, 2 out]
                }
                frame 37 {
                  n2998 = Match Pattern(string=w4025, regular expression=",") -> (before substring=w4024:string, after substring=w4023:string)  [unwired: 1 in, 2 out]
                  "bs" <- w4024
                  "as" <- w4023
                  n2999 = Concatenate Strings(w4024, w4023) -> (w4020:string)
                  n3000 = property on="Humidity before test 2" class="DigNum (strict)"("Caption.Text"=w4020) -> ()  [unwired: 2 in, 2 out]
                  n3001 = property on="Humidity before test" class="DigNum (strict)"("Caption.Text"=w4020) -> ()  [unwired: 2 in, 2 out]
                  n3002 = Concatenate Strings(w4020, "=" ("string")) -> (w4021:string)
                  n3003 = local write "S 38"(w4021) -> ()
                }
                frame 38 {
                  n3004 = Match Pattern(string=w4032, regular expression=",") -> (before substring=w4031:string, after substring=w4030:string)  [unwired: 1 in, 2 out]
                  "bs" <- w4031
                  "as" <- w4030
                  n3005 = Concatenate Strings(w4031, w4030) -> (w4027:string)
                  n3006 = property on="Humidity after test 2" class="DigNum (strict)"("Caption.Text"=w4027) -> ()  [unwired: 2 in, 2 out]
                  n3007 = Concatenate Strings(w4027, "=" ("string")) -> (w4029:string)
                  n3008 = property on="Humidity after test" class="DigNum (strict)"("Caption.Text"=w4027) -> ()  [unwired: 2 in, 2 out]
                  n3009 = local write "S 39"(w4029) -> ()
                }
                frame 39 {
                  n3010 = Match Pattern(string=w4039, regular expression=",") -> (before substring=w4038:string, after substring=w4037:string)  [unwired: 1 in, 2 out]
                  "bs" <- w4038
                  "as" <- w4037
                  n3011 = Concatenate Strings(w4038, w4037) -> (w4034:string)
                  n3012 = property on="Temperature before test 2" class="DigNum (strict)"("Caption.Text"=w4034) -> ()  [unwired: 2 in, 2 out]
                  n3013 = property on="Temperature before test" class="DigNum (strict)"("Caption.Text"=w4034) -> ()  [unwired: 2 in, 2 out]
                  n3014 = Concatenate Strings(w4034, "=" ("string")) -> (→"String 34":string)
                }
                frame 40 {
                  n3015 = Match Pattern(string=w4046, regular expression=",") -> (before substring=w4045:string, after substring=w4044:string)  [unwired: 1 in, 2 out]
                  "bs" <- w4045
                  "as" <- w4044
                  n3016 = Concatenate Strings(w4045, w4044) -> (w4041:string)
                  n3017 = property on="Temperature after test 2" class="DigNum (strict)"("Caption.Text"=w4041) -> ()  [unwired: 2 in, 2 out]
                  n3018 = Concatenate Strings(w4041, "=" ("string")) -> (→"String 35":string)
                  n3019 = property on="Temperature after test" class="DigNum (strict)"("Caption.Text"=w4041) -> ()  [unwired: 2 in, 2 out]
                }
                frame 41 {
                  n3020 = property on="AVP" class="DigNum (strict)"("Caption.Text"=w4050) -> ()  [unwired: 2 in, 2 out]
                  n3021 = property on="AVP 2" class="DigNum (strict)"("Caption.Text"=w4050) -> ()  [unwired: 2 in, 2 out]
                  n3022 = Concatenate Strings(w4050, "=" ("string")) -> (→"String 36":string)
                }
                frame 42 {
                  n3023 = property on="MWSD" class="DigNum (strict)"("Caption.Text"=w4053) -> ()  [unwired: 2 in, 2 out]
                  n3024 = property on="MWSD 2" class="DigNum (strict)"("Caption.Text"=w4053) -> ()  [unwired: 2 in, 2 out]
                  n3025 = Concatenate Strings(w4053, "=" ("string")) -> (→"String 37":string)
                }
                frame 43 {
                  n3026 = property on="HCF 2" class="DigNum (strict)"("Caption.Text"=w4056) -> ()  [unwired: 2 in, 2 out]
                  n3027 = property on="HCF" class="DigNum (strict)"("Caption.Text"=w4056) -> ()  [unwired: 2 in, 2 out]
                  n3028 = Concatenate Strings(w4056, "=" ("string")) -> (→"String 38":string)
                }
                frame 44 {
                  n3029 = Concatenate Strings(w4058, "=" ("string")) -> (→"String 39":string)
                  n3030 = property on="WS1.4 2" class="DigNum (strict)"("Caption.Text"=w4058) -> ()  [unwired: 2 in, 2 out]
                  n3031 = property on="WS1.4" class="DigNum (strict)"("Caption.Text"=w4058) -> ()  [unwired: 2 in, 2 out]
                }
                frame 45 {
                  n3032 = property on="Save Results" class="Bool (strict)"("Boolean Text.Text"=w4060) -> ()  [unwired: 2 in, 2 out]
                }
                frame 46 {
                  n3033 = local write "S 47"(w4061) -> ()
                }
                frame 47 {
                  n3034 = local write "S 48"(w4062) -> ()
                }
                frame 48 {
                  n3035 = local write "S 49"(w4063) -> ()
                }
                frame 49 {
                  n3036 = local write "S 50"(w4064) -> ()
                }
                frame 50 {
                  n3037 = local write "S 51"(w4065) -> ()
                }
                frame 51 {
                  n3038 = local write "S 52"(w4066) -> ()
                }
                frame 52 {
                  n3039 = local write "S 53"(w4067) -> ()
                }
                frame 53 {
                  n3040 = local write "S 54"(w4068) -> ()
                }
                frame 54 {
                  n3041 = local write "S 55"(w4069) -> ()
                }
                frame 55 {
                  n3042 = local write "S 56"(w4070) -> ()
                }
                frame 56 {
                  n3043 = local write "S 57"(w4071) -> ()
                }
                frame 57 {
                  n3044 = local write "S 58"(w4072) -> ()
                }
                frame 58 {
                  n3045 = local write "S 59"(w4073) -> ()
                }
                frame 59 {
                  n3046 = local write "S 60"(w4074) -> ()
                }
                frame 60 {
                  n3047 = local write "S 62"(w4075) -> ()
                }
                frame 61 {
                  n3048 = local write "S 63"(w4076) -> ()
                }
                frame 62 {
                  n3049 = local write "S 64"(w4077) -> ()
                }
                frame 63 {
                  n3050 = local write "S 65"(w4078) -> ()
                }
                frame 64 {
                  n3051 = local write "S 66"(w4079) -> ()
                }
                frame 65 {
                  n3052 = local write "S 67"(w4080) -> ()
                }
                frame 66 {
                  n3053 = local write "S 68"(w4081) -> ()
                }
                frame 67 {
                  n3054 = local write "S 69"(w4082) -> ()
                }
                frame 68 {
                  n3055 = local write "S 70"(w4083) -> ()
                }
                frame 69 {
                  n3056 = local write "S 71"(w4084) -> ()
                }
                frame 70 {
                  n3057 = local write "S 72"(w4085) -> ()
                }
                frame 71 {
                  n3058 = local write "S 73"(w4086) -> ()
                }
                frame 72 {
                  n3059 = local write "S 74"(w4087) -> ()
                }
                frame 73 {
                  n3060 = local write "S 75"(w4088) -> ()
                }
                frame 74 {
                  n3061 = local write "S 76"(w4089) -> ()
                }
                frame 75 {
                  n3062 = local write "S 77"(w4090) -> ()
                }
                frame 76 {
                  n3063 = local write "S 78"(w4091) -> ()
                }
                frame 77 {
                  n3064 = local write "S 79"(w4092) -> ()
                }
                frame 79 {
                  n3065 = property on="Sample Temperature ( °C )" class="XYGraph (strict)"("Y Scale.Name Label.Text"=w4093) -> ()  [unwired: 2 in, 2 out]
                }
                frame 80 {
                  n3066 = local write "S 81"(w4094) -> ()
                  n3067 = property on="Humidity ( %RH )" class="XYGraph (strict)"("Y Scale.Name Label.Text"=w4094) -> ()  [unwired: 2 in, 2 out]
                }
                frame 78 {
                  n3068 = property on="Air Temperature  ( °C )" class="XYGraph (strict)"("X Scale.Name Label.Text"=w4095) -> ()  [unwired: 2 in, 2 out]
                  n3069 = property on="Humidity ( %RH )" class="XYGraph (strict)"("X Scale.Name Label.Text"=w4095) -> ()  [unwired: 2 in, 2 out]
                  n3070 = property on="Sample Temperature ( °C )" class="XYGraph (strict)"("X Scale.Name Label.Text"=w4095) -> ()  [unwired: 2 in, 2 out]
                  n3071 = property on="Coefficient Of Friction" class="XYGraph (strict)"("X Scale.Name Label.Text"=w4095) -> ()  [unwired: 2 in, 2 out]
                }
                frame 81 {
                  n3072 = property on="Air Temperature  ( °C )" class="XYGraph (strict)"("Y Scale.Name Label.Text"=w4096) -> ()  [unwired: 2 in, 2 out]
                }
                frame 82 {
                  n3073 = local write "S 84"(w4097) -> ()
                }
                frame 83 {
                  n3074 = local write "S 85"(w4098) -> ()
                }
                frame 84 {
                  n3075 = local write "S 86"(w4099) -> ()
                }
                frame 85 {
                  n3076 = local write "S 87"(w4100) -> ()
                }
                frame 86 {
                  n3077 = local write "S 88"(w4101) -> ()
                }
                frame 87 {
                }
                frame 88 {
                  n3078 = local write "S 90"(w4103) -> ()
                }
                frame 89 {
                  n3079 = local write "S 91"(w4104) -> ()
                }
                frame 90 {
                  n3080 = local write "S 92"(w4105) -> ()
                }
                frame 91 {
                  n3081 = local write "S 93"(w4106) -> ()
                }
                frame 92 {
                  n3082 = local write "S 94"(w4107) -> ()
                }
                frame 93 {
                  n3083 = local write "S 95"(w4108) -> ()
                }
                frame 94 {
                  n3084 = local write "S 96"(w4109) -> ()
                }
                frame 95 {
                  n3085 = local write "S 97"(w4110) -> ()
                }
                frame 96 {
                  n3086 = local write "S 98"(w4111) -> ()
                }
                frame 97 {
                  n3087 = local write "S 99"(w4112) -> ()
                }
                frame 98 {
                  n3088 = local write "S 100"(w4113) -> ()
                }
                frame 99 {
                  n3089 = local write "S 101"(w4114) -> ()
                }
                frame 100 {
                  n3090 = local write "S 102"(w4115) -> ()
                }
                frame 101 {
                  n3091 = local write "S 103"(w4116) -> ()
                }
                frame 102 {
                  n3092 = local write "S 104"(w4117) -> ()
                }
                frame 103 {
                  n3093 = local write "S 105"(w4118) -> ()
                }
                frame 104 {
                  n3094 = local write "S 106"(w4119) -> ()
                }
                frame 105 {
                }
                frame 106 {
                  n3095 = property on="OK Button 17" class="Bool (strict)"("Boolean Text.Text"=w4120) -> ()  [unwired: 2 in, 2 out]
                }
                frame 107 {
                  n3096 = property on="OK Button 16" class="Bool (strict)"("Boolean Text.Text"=w4121) -> ()  [unwired: 2 in, 2 out]
                }
                frame 108 {
                  n3097 = property on="TITTLE" class="Str"("Caption.Text"=w4122) -> ()  [unwired: 2 in, 2 out]
                }
                frame 109 {
                  "String 30" <- w4123
                }
                frame 110 {
                  n3098 = property on="Test Date" class="Str"("Caption.Text"=w4124) -> ()  [unwired: 2 in, 2 out]
                  "String 31" <- w4124
                }
                frame 111 {
                  n3099 = property on="Sample ID" class="Str"("Caption.Text"=w4125) -> ()  [unwired: 2 in, 2 out]
                  "String 32" <- w4125
                }
                frame 112 {
                  n3100 = property on="Tested by" class="Str"("Caption.Text"=w4126) -> ()  [unwired: 2 in, 2 out]
                  "String 33" <- w4126
                }
                frame 113 {
                  n3101 = property on="System Configured Printers 2" class="Arr (strict)"("Caption.Text"=w4127) -> ()  [unwired: 2 in, 2 out]
                }
                frame 114 {
                  n3102 = property on="Selected Printer" class="Str"("Caption.Text"=w4128) -> ()  [unwired: 2 in, 2 out]
                }
                frame 115 {
                  n3103 = property on="Select Printer 3" class="DigNum (strict)"("Caption.Text"=w4129) -> ()  [unwired: 2 in, 2 out]
                }
                frame 116 {
                  n3104 = property on="Print" class="Bool (strict)"("Boolean Text.Text"=w4130) -> ()  [unwired: 2 in, 2 out]
                }
                frame 117 {
                  "String 41" <- w4131
                }
                frame 118 {
                  n3105 = property on="tested by" class="Str"("Caption.Text"=w4132) -> ()  [unwired: 2 in, 2 out]
                }
                frame 119 {
                }
                frame 120 {
                  n3106 = property on="Export" class="Bool (strict)"("Boolean Text.Text"=w4133) -> ()  [unwired: 2 in, 2 out]
                }
                frame 121 {
                  n3107 = property on="TEMP INTERCEPT:" class="DigNum (strict)"("Caption.Text"=w4134) -> ()  [unwired: 2 in, 2 out]
                }
                frame 122 {
                  n3108 = property on="AIR TEMP INTERCEPT:" class="DigNum (strict)"("Caption.Text"=w4135) -> ()  [unwired: 2 in, 2 out]
                }
                frame 123 {
                  n3109 = property on="Select File Type" class="Enum (strict)"("Caption.Text"=w4136) -> ()  [unwired: 2 in, 2 out]
                }
                frame 124 {
                  n3110 = property on="s.NO" class="Str"("Caption.Text"=w4137) -> ()  [unwired: 2 in, 2 out]
                  "String 45" <- w4137
                }
                frame 125 {
                  n3111 = property on="trip1 8" class="Bool (strict)"("Boolean Text.Text"=w4138) -> ()  [unwired: 2 in, 2 out]
                }
